vi "CE Get Measurement Path.vi"(8 "Template line":i32, 11 "Measurement template file":path=path "D:/martin/WAC/WACsw - github/control_software/Filter function meter/Template/Example of FF meter template.xlsx") -> (0 "Measurement path as string":string, 3 "Measurement path":path)   [LabVIEW 2020]
doc: "Generate paths for CE measurement data based on the CE template file."
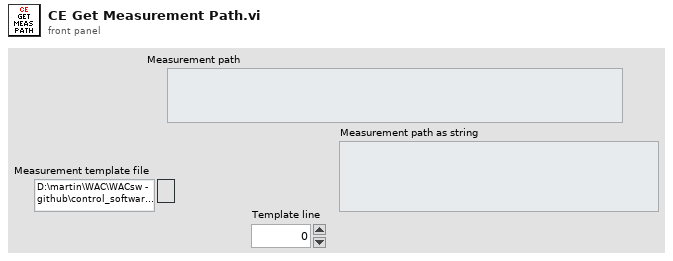
[diagram p1: front panel]
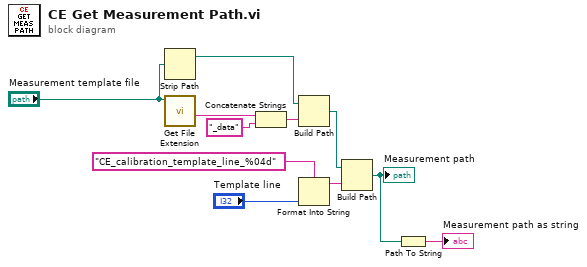
[diagram p0: block diagram]
diagram:
  n1 = Strip Path(path="Measurement template file") -> (stripped path=w9:path)  [unwired: 1 out]
  n2 = call <vilib>:"Get File Extension.vi"("file"="Measurement template file") -> ("filename without extension"=w7:string)  [unwired: 6 in, 4 out]
  n3 = Concatenate Strings(w7, "_data" ("string")) -> (w5:string)
  n4 = Build Path(base path=w9, name or relative path=w5) -> (appended path=w8:path)
  n5 = Format Into String(format string="CE_calibration_template_line_%04d", "Template line") -> (resulting string=w3:string)  [unwired: 2 in, 1 out]
  n6 = Build Path(base path=w8, name or relative path=w3) -> (appended path=w2:path)
  "Measurement path" <- w2
  n7 = Path To String(path=w2) -> (string=→"Measurement path as string":string)
